vi "AT Set Enum String A.vi"(8 "error in (no error)":errorcluster, 9 "String":string, 10 "Feature":string, 11 "Handle":i32) -> (0 "error out":errorcluster, 3 "Status":i32)   [LabVIEW 2019]
doc: "Set Enum String\n\nOutput:\n I32 Status\n\nInput:\n I32 Handle\n String Feature\n String String\n\nThis function directly sets the current value of the specified enumerated feature. The String parameter must be one of the allowed values for the feature and must be currently available."
uses:
  atcoreA.dll
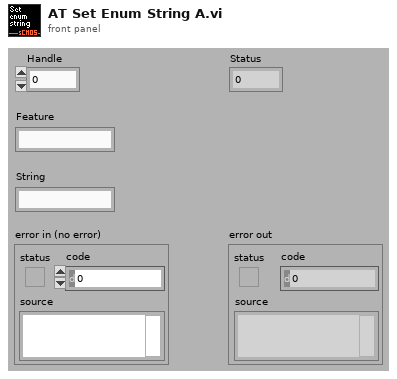
[diagram p1: front panel]
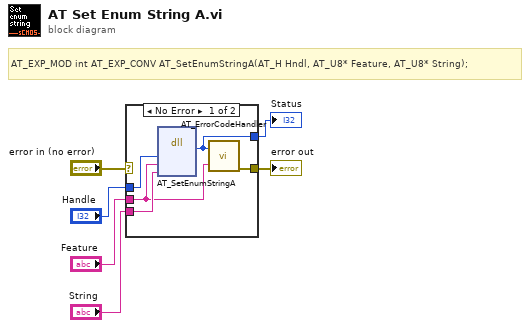
[diagram p0: block diagram]
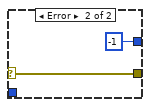
[diagram p2: hidden frame]
diagram:
  # "AT_EXP_MOD int AT_EXP_CONV AT_SetEnumStringA(AT_H Hndl, AT_U8* Feature, AT_U8* String);"
  n1 = case shown="No Error" "error in (no error)" {
    selector: "error in (no error)" -> [_ w13]
    tunnel: [w8 -1 ("return type")] -> w6
    tunnel: "Handle" -> [w11 _]
    tunnel: "Feature" -> [w7 _]
    tunnel: "String" -> [w10 _]
    tunnel: [w9 w13] -> w1
    frame No Error {
      n2 = dll-call lib="atcoreA.dll" fn="AT_SetEnumStringA"("Handle"=w11, "Feature"=w7, "String"=w10) -> ("Status"=w8:i32)  [unwired: 6 in, 2 out]
      n3 = call "AT_ErrorCodeHandler.vi"("Error"=w8, "Feature Name"=w7) -> ("error out"=w9:errorcluster)  [unwired: 5 in]
    }
    frame Error {
    }
  }
  "Status" <- w6
  "error out" <- w1
